vi "Read Position.vi"(5 "Username":string, 6 "Password":string, 7 "Address":string, 8 "Error In":errorcluster) -> (0 "Error Out":errorcluster)   [LabVIEW 2018, in "Tests.lvlib" / "SFTP File.lvlib"]
uses:
  SFTP File.lvlib
  src/Toolkit/API/SFTP File/API/Typedefs/Flags.ctl
  src/Toolkit/API/SFTP File/SFTP File.lvclass/SFTP File.ctl
  src/Toolkit/API/SFTP/SFTP.lvclass/SFTP.ctl
  src/Toolkit/API/SFTP/Utility/Read Shared Library.vi
  src/Toolkit/API/Session/Utility/Read Shared Library.vi
  src/Toolkit/Support/Check Status.vi
  <vilib>/addons/_JKI Toolkits/Caraya/classes/Test/Test.lvclass
  <vilib>/addons/_JKI Toolkits/Caraya/classes/Assert/Assert.lvclass
  src/Toolkit/API/SFTP File/SFTP File.lvclass
  src/Toolkit/API/SFTP/SFTP.lvclass
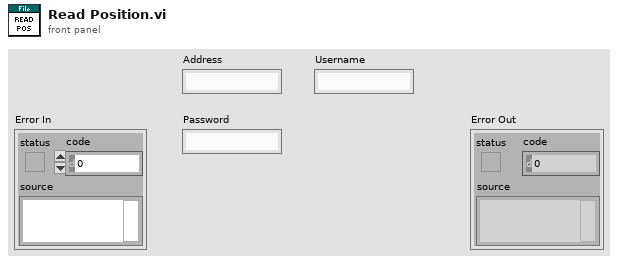
[diagram p1: front panel]
types:
  T1 = typedef "Toolkit.lvlib/SFTP File.lvclass/Flags.ctl" = cluster{"Read":bool, "Write":bool, "Append":bool, "Create":bool, "Truncate":bool, "Exclude":bool}
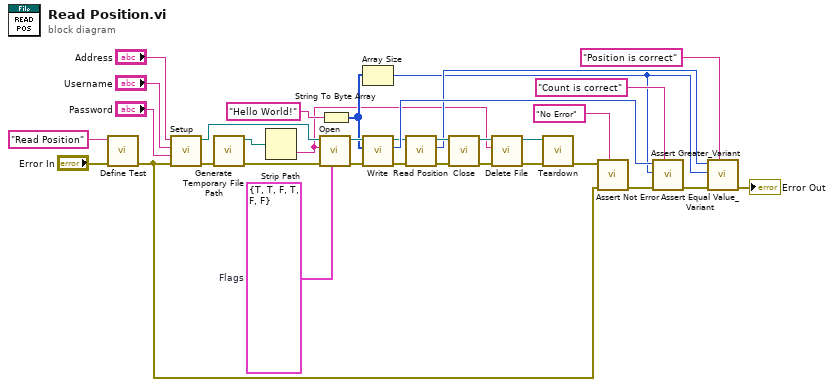
[diagram p0: block diagram]
diagram:
  w13 = T1 {"Read"=TRUE, "Write"=TRUE, "Append"=FALSE, "Create"=TRUE, "Truncate"=FALSE, "Exclude"=FALSE}  # Flags
  n1 = call <vilib>:"Define Test.vi"("error in (no error)"="Error In", "Label (VI Title)"="Read Position") -> ("error out"=w25:errorcluster)  [unwired: 9 in]
  n2 = call "Setup.vi"("Error In"=w25, "Password"="Password", "Username"="Username", "Address"="Address") -> ("Error Out"=w21:errorcluster, "SFTP"=w23:refnum<class "SFTP.lvclass">)  [unwired: 6 in]
  n3 = call <vilib>:"Generate Temporary File Path.vi"("error in (no error)"=w21) -> ("error out"=w20:errorcluster, "Unique Temporary File Path"=w19:path)  [unwired: 9 in]
  n4 = Strip Path(path=w19) -> (name=w1:string)  [unwired: 1 out]
  n5 = call "Open.vi"("Flags"=w13, "Error In"=w20, "Remote Path"=w1, "SFTP"=w23) -> ("Error Out"=w16:errorcluster, "SFTP File"=w18:refnum<class "SFTP File.lvclass">)  [unwired: 6 in]
  n6 = String To Byte Array(string="Hello World!") -> (unsigned byte array=w14:u8[])
  n7 = Array Size(array=w14) -> (size(s)=w6:i32)
  n8 = call "Write.vi"("Error In"=w16, "Data"=w14, "SFTP File In"=w18) -> ("Error Out"=w9:errorcluster, "Count"=w17:i64, "SFTP File Out"=w12:refnum<class "SFTP File.lvclass">)  [unwired: 6 in]
  n9 = call "Read Position.vi"("Error In"=w9, "SFTP File In"=w12) -> ("Error Out"=w10:errorcluster, "Position"=w7:u64, "SFTP File Out"=w11:refnum<class "SFTP File.lvclass">)  [unwired: 7 in]
  n10 = call "Close.vi"("Error In"=w10, "SFTP File"=w11) -> ("Error Out"=w3:errorcluster, "SFTP"=w22:refnum<class "SFTP.lvclass">)  [unwired: 8 in]
  n11 = call "Delete File.vi"("Error In"=w3, "Remote Path"=w1, "SFTP In"=w22) -> ("Error Out"=w2:errorcluster, "SFTP Out"=w4:refnum<class "SFTP.lvclass">)  [unwired: 7 in]
  n12 = call "Teardown.vi"("Error In"=w2, "SFTP"=w4) -> ("Error Out"=w24:errorcluster)  [unwired: 9 in]
  n13 = call <vilib>:"Assert Not Error.vi"("Label"="No Error", "error in (no error)"=w25, "Not Error?"=w24) -> ("error out"=w31:errorcluster)  [unwired: 8 in]
  n14 = call <vilib>:"Assert Greater_Variant.vi"("Label"="Count is correct", "error in (no error)"=w31, "Y"=w6, "X"=w17) -> ("error out"=w30:errorcluster)  [unwired: 7 in]
  n15 = call <vilib>:"Assert Equal Value_Variant.vi"("Label"="Position is correct", "error in (no error)"=w30, "Y"=w6, "X"=w7) -> ("error out"=→"Error Out":errorcluster)  [unwired: 7 in]
